vi "Keithley 6517A DCI Config.vi"(0 "GPIB address":string="27", 1 "integration time (0:auto)":u16(ring) items=["automatic NPLC", "automatic NPLC once", "set to minimum NPLC", "set to maximum NPLC", "set NPLC value"], 2 "NPLC value":dbl=1.0 min=0.01 max=10.0 step=0.01 format="%.2f", 3 "range (auto:0)":u16(ring) items=["autorange", "autorange once", "set min range", "set max range", "set range value"], 4 "range value (amps)":dbl=0.02 min=2e-11 max=0.02 format="%^.2e", 5 "error in":T1, 6 "damping":bool, 7 "resolution (5.5 digits:4)":u16(ring)=3 items=["auto resolution", "auto resolution once", "3.5 digits", "4.5 digits", "5.5 digits", "6.5 digits"], 8 "reference (off:0)":u16(ring) items=["off", "set reference value"], 9 "digital filter type (off:0)":u16(ring) items=["None", "Averaging", "Advanced"], 10 "reference value (amps)":dbl min=-0.02 max=0.02 format="%^.2e", 11 "dig. filter count":i16=10 min=1 max=100 step=1, 12 "Median":u16(ring) items=["Off", "On"], 13 "Median Rank":i16=1 min=1 max=5 step=1, 14 "filter type control (Moving:0)":u16(ring) items=["Moving", "Repeat"], 15 "noise tolerance (%)":dbl=1.0 min=1.0 max=100.0 step=0.01 format="%.3f") -> (19 "error out":T1)   [LabVIEW 2013]
doc: "This VI is used to configure the settings for the DC current measurements. The instrument can be in any mode when this VI is run. The settings will go into effect and the instrument will go into the DC current mode."
panel:
  # "On\nOff"
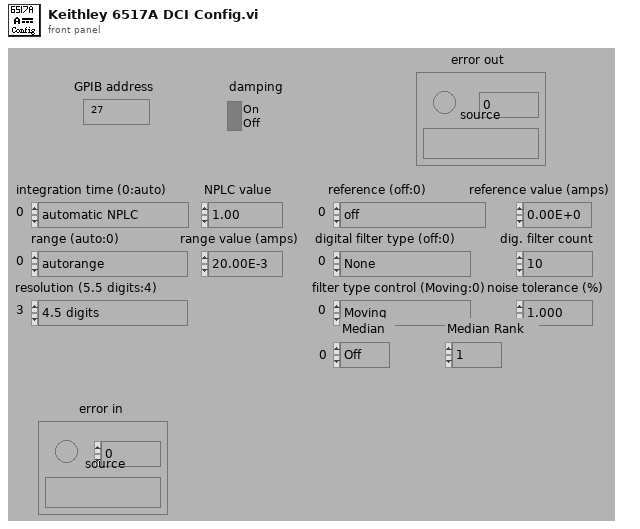
[diagram p1: front panel]
types:
  T1 = cluster{"error":bool, "code":i32, "source":string}
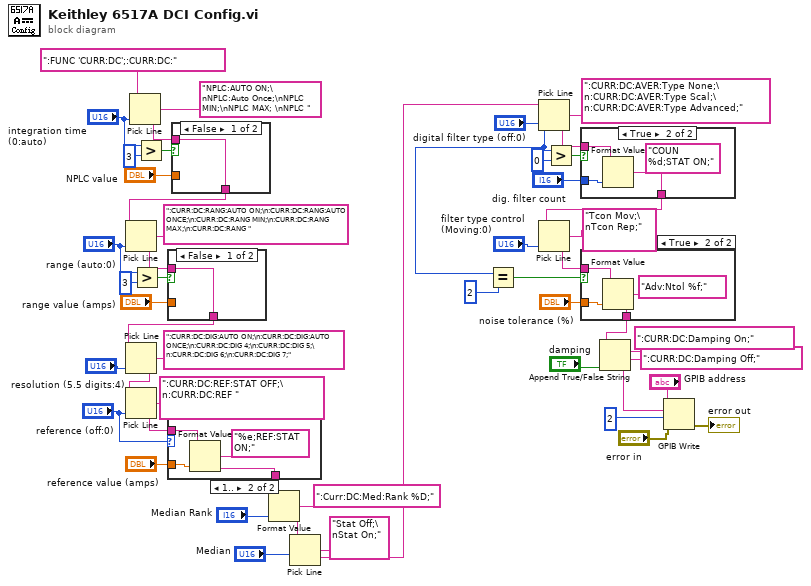
[diagram p0: block diagram]
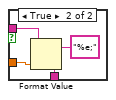
[diagram p5: hidden frame]
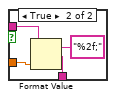
[diagram p6: hidden frame]
diagram:
  n1 = Pick Line(string ("")=":FUNC 'CURR:DC';:CURR:DC:", multi-line string="NPLC:AUTO ON;\nNPLC:Auto Once;\nNPLC MIN;\nNPLC MAX; \nNPLC ", line index="integration time (0:auto)") -> (output string=w17:string)
  n2 = Greater?(x="range (auto:0)", y=3) -> (0:w45:bool)
  n3 = Greater?(x="integration time (0:auto)", y=3) -> (0:w47:bool)
  n4 = case shown="False" w47 {
    tunnel: "NPLC value" -> [_ w55]
    tunnel: [w52 w53] -> w16
    tunnel: w17 -> [w52 w54]
    frame False {
    }
    frame True {
      n5 = Format Value(string ("")=w54, format string="%2f;", value (0)=w55) -> (output string=w53:string)
    }
  }
  n6 = Pick Line(string ("")=w16, multi-line string=":CURR:DC:RANG:AUTO ON;\n:CURR:DC:RANG:AUTO ONCE;\n:CURR:DC:RANG MIN;\n:CURR:DC:RANG MAX;\n:CURR:DC:RANG ", line index="range (auto:0)") -> (output string=w46:string)
  n7 = case shown="False" w45 {
    tunnel: "range value (amps)" -> [_ w60]
    tunnel: w46 -> [w57 w59]
    tunnel: [w57 w58] -> w15
    frame False {
    }
    frame True {
      n8 = Format Value(string ("")=w59, format string="%e;", value (0)=w60) -> (output string=w58:string)
    }
  }
  n9 = Pick Line(string ("")=w15, multi-line string=":CURR:DC:DIG:AUTO ON;\n:CURR:DC:DIG:AUTO ONCE;\n:CURR:DC:DIG 4;\n:CURR:DC:DIG 5;\n:CURR:DC:DIG 6;\n:CURR:DC:DIG 7;", line index="resolution (5.5 digits:4)") -> (output string=w14:string)
  n10 = Pick Line(string ("")=w14, multi-line string=":CURR:DC:REF:STAT OFF;\n:CURR:DC:REF ", line index="reference (off:0)") -> (output string=w38:string)
  n11 = case shown="1.." "reference (off:0)" {
    tunnel: "reference value (amps)" -> [_ w66]
    tunnel: w38 -> [w62 w65]
    tunnel: [w62 w63] -> w13
    frame ..0 {
    }
    frame 1.. {
      n12 = Format Value(string ("")=w65, format string="%e;REF:STAT ON;", value (0)=w66) -> (output string=w63:string)
    }
  }
  n13 = Format Value(string ("")=w13, format string=":Curr:DC:Med:Rank %D;", value (0)="Median Rank") -> (output string=w12:string)
  n14 = Pick Line(string ("")=w12, multi-line string="Stat Off;\nStat On;", line index="Median") -> (output string=w9:string)
  n15 = Equal?(x="digital filter type (off:0)", y=2) -> (x = y?=w8:bool)
  n16 = Pick Line(string ("")=w9, multi-line string=":CURR:DC:AVER:Type None;\n:CURR:DC:AVER:Type Scal;\n:CURR:DC:AVER:Type Advanced;", line index="digital filter type (off:0)") -> (output string=w34:string)
  n17 = Greater?(x="digital filter type (off:0)", y=0) -> (0:w31:bool)
  n18 = case shown="True" w31 {
    tunnel: "dig. filter count" -> [_ w71]
    tunnel: w34 -> [w67 w70]
    tunnel: [w67 w69] -> w25
    frame False {
    }
    frame True {
      n19 = Format Value(string ("")=w70, format string="COUN %d;STAT ON;", value (0)=w71) -> (output string=w69:string)
    }
  }
  n20 = Pick Line(string ("")=w25, multi-line string="Tcon Mov;\nTcon Rep;", line index="filter type control (Moving:0)") -> (output string=w28:string)
  n21 = case shown="True" w8 {
    tunnel: "noise tolerance (%)" -> [_ w76]
    tunnel: w28 -> [w72 w75]
    tunnel: [w72 w74] -> w21
    frame False {
    }
    frame True {
      n22 = Format Value(string ("")=w75, format string="Adv:Ntol %f;", value (0)=w76) -> (output string=w74:string)
    }
  }
  n23 = Append True/False String(1:"damping", 2:":CURR:DC:Damping Off;", 3:":CURR:DC:Damping On;", 4:w21) -> (0:w4:string)
  n24 = GPIB Write(0:"GPIB address", 1:w4, 2:2, 3:"error in") -> (6:→"error out":errorcluster)  [unwired: 1 in, 1 out]
